vi "SimpleReadWrite.vi"() -> ()   [LabVIEW 2016]
uses:
  PLC_Attributes.ctl
panel:
  out "Error Codes":string="PLCTAG_STATUS_OK\nPLCTAG_STATUS_OK\nPLCTAG_STATUS_OK\nPLCTAG_STATUS_OK\nPLCTAG_STATUS_OK\nPLCTAG_STATUS_OK"
  out "new tag value read":sgl=3.66
  in  "new value to write":sgl=3.66
  out "original tag value read":sgl=15.236
  in  "PLC Attributes":T1={"protocol"="ab-eip", "path"="1,0", "gatewayIP"="192.168.1.40", "cpu"="lgx", "element size"="4", "element count"="1", "tag name"="Enter your tag name here", "debug level"="NONE"}
  # "Simple Example that reads a float from a tag, writes a new value, then reads that value."
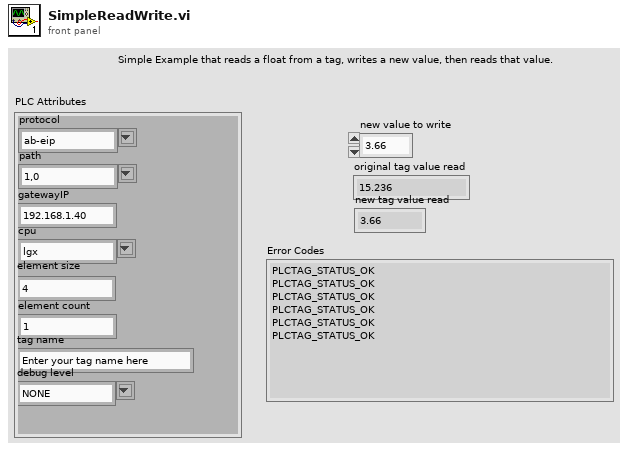
[diagram p1: front panel]
types:
  T1 = typedef "PLC_Attributes.ctl" = cluster{"protocol":string, "path":string, "gatewayIP":string, "cpu":string, "element size":string, "element count":string, "tag name":string, "debug level":string}
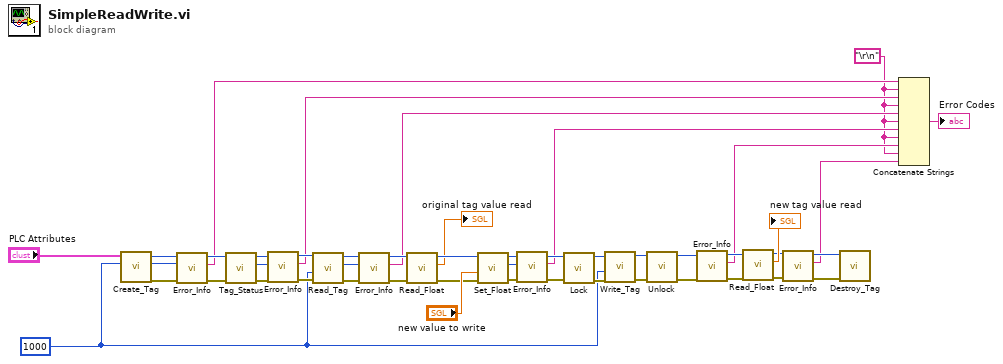
[diagram p0: block diagram]
diagram:
  w3 = "\r\n"
  w9 = 1000 ("timeout")
  n1 = call "Create_Tag.vi"("timeout"=w9, "PLC Attributes"="PLC Attributes") -> ("error out"=w45:errorcluster, "error code"=w46:i32, "handle"=w47:i32)  [unwired: 7 in]
  n2 = call "Error_Info.vi"("error in (no error)"=w45, "errorcode"=w46, "tag handle"=w47) -> ("error out"=w43:errorcluster, "error description"=w8:string, "tag handle out"=w44:i32)  [unwired: 6 in]
  n3 = call "Tag_Status.vi"("error in (no error)"=w43, "tag handle"=w44) -> ("error out"=w42:errorcluster, "error code"=w41:i32, "tag handle out"=w40:i32)  [unwired: 7 in]
  n4 = call "Error_Info.vi"("error in (no error)"=w42, "errorcode"=w41, "tag handle"=w40) -> ("error out"=w38:errorcluster, "error description"=w7:string, "tag handle out"=w39:i32)  [unwired: 6 in]
  n5 = call "Read_Tag.vi"("error in (no error)"=w38, "timeout"=w9, "tag handle"=w39) -> ("error out"=w37:errorcluster, "error code"=w36:i32, "tag handle out"=w35:i32)  [unwired: 6 in]
  n6 = call "Error_Info.vi"("error in (no error)"=w37, "errorcode"=w36, "tag handle"=w35) -> ("error out"=w21:errorcluster, "error description"=w6:string, "tag handle out"=w22:i32)  [unwired: 6 in]
  n7 = call "Read_Float.vi"("error in (no error)"=w21, "tag handle"=w22) -> ("error out"=w19:errorcluster, "tag value"=→"original tag value read":sgl, "tag handle out"=w20:i32)  [unwired: 7 in]
  n8 = call "Set_Float.vi"("error in (no error)"=w19, "value"="new value to write", "tag handle"=w20) -> ("error out"=w30:errorcluster, "error code"=w32:i32, "tag handle out"=w31:i32)  [unwired: 6 in]
  n9 = call "Error_Info.vi"("error in (no error)"=w30, "errorcode"=w32, "tag handle"=w31) -> ("error out"=w17:errorcluster, "error description"=w5:string, "tag handle out"=w18:i32)  [unwired: 6 in]
  n10 = call "Lock.vi"("error in (no error)"=w17, "tag handle"=w18) -> ("error out"=w15:errorcluster, "tag handle out"=w16:i32)  [unwired: 7 in, 1 out]
  n11 = call "Write_Tag.vi"("error in (no error)"=w15, "timeout"=w9, "tag handle"=w16) -> ("error out"=w13:errorcluster, "tag handle out"=w14:i32)  [unwired: 6 in, 1 out]
  n12 = call "Unlock.vi"("error in (no error)"=w13, "tag handle"=w14) -> ("error out"=w11:errorcluster, "tag handle out"=w12:i32)  [unwired: 7 in, 1 out]
  n13 = call "Error_Info.vi"("error in (no error)"=w11, "tag handle"=w12) -> ("error out"=w29:errorcluster, "error description"=w4:string, "tag handle out"=w28:i32)  [unwired: 7 in]
  n14 = call "Read_Float.vi"("error in (no error)"=w29, "tag handle"=w28) -> ("error out"=w26:errorcluster, "tag value"=→"new tag value read":sgl, "tag handle out"=w25:i32)  [unwired: 7 in]
  n15 = call "Error_Info.vi"("error in (no error)"=w26, "tag handle"=w25) -> ("error out"=w23:errorcluster, "error description"=w2:string, "tag handle out"=w24:i32)  [unwired: 7 in]
  n16 = call "Destroy_Tag.vi"("error in (no error)"=w23, "tag handle"=w24) -> ()  [unwired: 8 in, 2 out]
  n17 = Concatenate Strings(w8, w3, w7, w3, w6, w3, w5, w3, w4, w3, w2) -> (→"Error Codes":string)
